vi "Begin.vi"() -> (0 "error out":errorcluster)   [LabVIEW 2014]
doc: "Called before other user functions, this VI is expected to open initial I/O refnums, load in file data, and do all program initialization. Notice that the <B>error out</B> terminal is simply used for data flow. Wiring it to other structures or subVIs ensures that this VI runs first."
uses:
  <vilib>/Rock Robotics/WPI/SafetyOutput/WPI_SafetyOutputConfigMenu.ctl
  Robot Global Data.vi
  <vilib>/Rock Robotics/WPI/DriverStation/WPI_DriverStationRobotMode2.ctl
  <vilib>/Rock Robotics/WPI/Joystick/WPI_JoystickDeviceEnum.ctl
  <vilib>/Rock Robotics/SystemInterfaces/DIO/FPGA_DIOPWMChannel.ctl
  <vilib>/Rock Robotics/SystemInterfaces/AI/FPGA_AIGyroChannel.ctl
  <vilib>/Rock Robotics/SystemInterfaces/Typedef/FPGA_TypedefAnalogModuleForGyro.ctl
  <vilib>/Rock Robotics/WPI/Counter/WPI_CounterDigitalInputToDigitalSource.vi
  <vilib>/Rock Robotics/SystemInterfaces/DIO/FPGA_DIOChannel.ctl
  <vilib>/Rock Robotics/WPI/Encoder/WPI_EncoderType.ctl
  <vilib>/Rock Robotics/SystemInterfaces/DIO/FPGA_DIORelayChannel.ctl
  <vilib>/Rock Robotics/WPI/Relay/WPI_RelayDirection.ctl
  <vilib>/Rock Robotics/SystemInterfaces/Typedef/FPGA_TypedefDigitalModule.ctl
  <vilib>/Rock Robotics/WPI/MotorControl/WPI_MotorControlOpen Victor.vi
  <vilib>/Rock Robotics/WPI/Relay/WPI_RelayValue.ctl
  <vilib>/Rock Robotics/WPI/RobotDrive/WPI_RobotDriveOpen4MotorWithTalon.vi
  <vilib>/Rock Robotics/SystemInterfaces/AI/FPGA_AIChannel.ctl
panel:
  out "error out 7":errorcluster
  out "error out 6":errorcluster
  out "error out 5":errorcluster
  out "error out 4":errorcluster
  out "error out 3":errorcluster
  out "error out 2":errorcluster
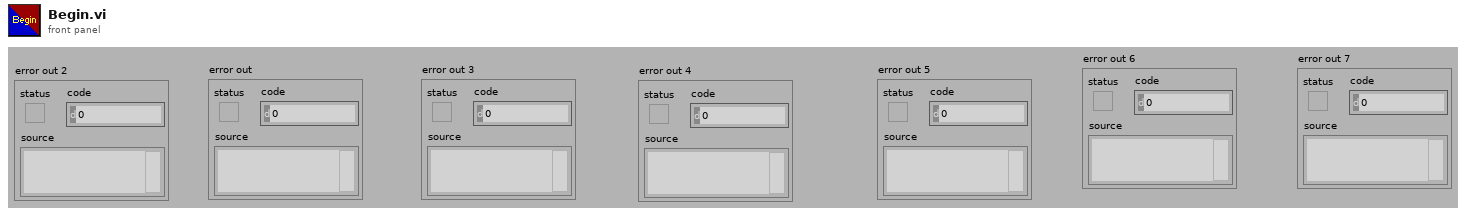
[diagram p1: front panel]
types:
  T1 = typedef "FPGA_AIChannel.ctl" = enum8{"AI 1", "AI 2", "AI 3", "AI 4", "AI 5", "AI 6", "AI 7", "AI 8", "Invalid"}
  T2 = typedef "FPGA_DIOChannel.ctl" = enum8{"DIO 1", "DIO 2", "DIO 3", "DIO 4", "DIO 5", "DIO 6", "DIO 7", "DIO 8", "DIO 9", "DIO 10", "DIO 11", "DIO 12", "DIO 13", "DIO 14", "Invalid"}
  T3 = typedef "WPI_RelayValue.ctl" = enum16{"Off", "On", "Forward", "Reverse"}
  T4 = typedef "FPGA_TypedefDigitalModule.ctl" = enum16{"Digital Module 1", "Digital Module 2"}
  T5 = typedef "FPGA_DIORelayChannel.ctl" = enum8{"Relay 1", "Relay 2", "Relay 3", "Relay 4", "Relay 5", "Relay 6", "Relay 7", "Relay 8", "Invalid"}
  T6 = typedef "FPGA_DIOPWMChannel.ctl" = enum8{"PWM 1", "PWM 2", "PWM 3", "PWM 4", "PWM 5", "PWM 6", "PWM 7", "PWM 8", "PWM 9", "PWM 10", "Invalid"}
  T7 = typedef "WPI_RelayDirection.ctl" = enum16{"Both directions", "Forward only", "Reverse only"}
  T8 = typedef "WPI_EncoderType.ctl" = enum16{"1x", "2x", "4x"}
  T9 = typedef "WPI_JoystickDeviceEnum.ctl" = enum16{"USB 1", "USB 2", "USB 3", "USB 4", "Kinect 1", "Kinect 2"}
  T10 = typedef "FPGA_TypedefAnalogModuleForGyro.ctl" = enum16{"Analog Module 1"}
  T11 = typedef "FPGA_AIGyroChannel.ctl" = enum8{"AI 1", "AI 2", "Invalid"}
  T12 = typedef "WPI_DriverStationRobotMode2.ctl" = enum16{"Autonomous Disabled", "Autonomous Enabled", "Teleop Disabled", "Teleop Enabled", "Timeout", "Finish", "Test Disabled", "Test Enabled"}
  T13 = typedef "WPI_SafetyOutputConfigMenu.ctl" = enum16{"Enable", "Disable"}
  T14 = typedef "WPI_AnalogChannelDevRef.ctl" = cluster{"DevStatus":errorcluster, "Analog Module":T15, "Analog Channel":T1}
  T15 = typedef "FPGA_TypedefAnalogModule.ctl" = enum16{"Analog Module 1", "Analog Module 2"}
  T16 = typedef "WPI_DigitalInputDevRef.ctl" = cluster{"DevStatus":errorcluster, "DIO Channel":T2, "Digital Module":T4}
  T17 = typedef "WPI_JoystickDevRef.ctl" = cluster{"Device":T9}
  T18 = typedef "WPI_MotorControlDeviceRef.ctl" = cluster{"DeviceStatus":errorcluster, "Type":enum16{"PWM", "CAN"}, "PWM":cluster{"Digital Module":T4, "PWM Channel":T6, "DeadBand":T19}, "CAN":cluster{"Device Number":u8, "Control Mode":T20, "Semaphore":T21, "Max Vout":dbl}, "Invert":bool, "TransformRef":T22, "InvTransformRef":T22}
  T19 = typedef "WPI_PWMDeadband.ctl" = cluster{"Name":string, "maxPositivePwm":i32, "minPositivePwm":i32, "centerPwm":i32, "maxNegativePwm":i32, "minNegativePwm":i32, "angularRange":u16}
  T20 = typedef "WPI_CANJaguar_ControlMode.ctl" = enum8{"Percent VBus", "Current", "Speed", "Position", "Voltage"}
  T21 = typedef "Semaphore RefNum" = refnum<k1>
  T22 = typedef "WPI_PWMTransform_ConPane.ctl" = refnum<vi>
  T23 = typedef "WPI_RelayDevRef.ctl" = cluster{"DevStatus":errorcluster, "Relay Channel":T5, "Digital Module":T4, "Relay Direction":T7}
  T24 = typedef "FPGA_CounterEncoderSourceConvertionLVSourceType.ctl" = cluster{"DevStatus":errorcluster, "AnalogTriggerMode?":bool, "DigitalMode":cluster{"Digital Module":T4, "DIO Channel":T25}, "AnalogTriggerMode":cluster{"AnalogTriggerIndex":T26, "OutputType":T27}}
  T25 = typedef "FPGA_DIODigitalSourceChannel.ctl" = enum8{"DIO 1", "DIO 2", "DIO 3", "DIO 4", "DIO 5", "DIO 6", "DIO 7", "DIO 8", "DIO 9", "DIO 10", "DIO 11", "DIO 12", "DIO 13", "DIO 14", "Disabled"}
  T26 = typedef "FPGA_AnalogTriggerIndex.ctl" = enum8{"Trig 0", "Trig 1", "Trig 2", "Trig 3", "Trig 4", "Trig 5", "Trig 6", "Trig 7", "Invalid"}
  T27 = typedef "FPGA_AnalogTriggerOutType.ctl" = enum16{"InWindow", "TriggerState", "Rising", "Falling"}
  T28 = typedef "WPI_RobotDriveDevRef.ctl" = cluster{"DevStatus":errorcluster, "Motors[]":T18[], "Square Inputs":bool, "Max Output":dbl, "Isochronous":bool}
  T29 = typedef "WPI_CompressorDevRef.ctl" = cluster{"DevStatus":errorcluster, "DigitalInputDevRef":T16, "RelayDevRef":T23}
  T30 = typedef "WPI_GyroDevRef.ctl" = cluster{"DevStatus":errorcluster, "Analog Module":T15, "Analog Channel":T1, "Offset":dbl, "Gain (VoltsPerDegree/Second)":dbl}
  T31 = typedef "WPI_EncoderDevRef.ctl" = cluster{"DevStatus":errorcluster, "EncoderIndex":T32, "CounterIndex":T33, "DistancePerCount":dbl, "Decoding Type":T8}
  T32 = typedef "FPGA_EncoderIdx.ctl" = enum8{"Enc 0", "Enc 1", "Enc 2", "Enc 3", "Invalid"}
  T33 = typedef "FPGA_CounterCtrSystemIndex.ctl" = enum8{"Ctr 0", "Ctr 1", "Ctr 2", "Ctr 3", "Ctr 4", "Ctr 5", "Ctr 6", "Ctr 7", "Invalid"}
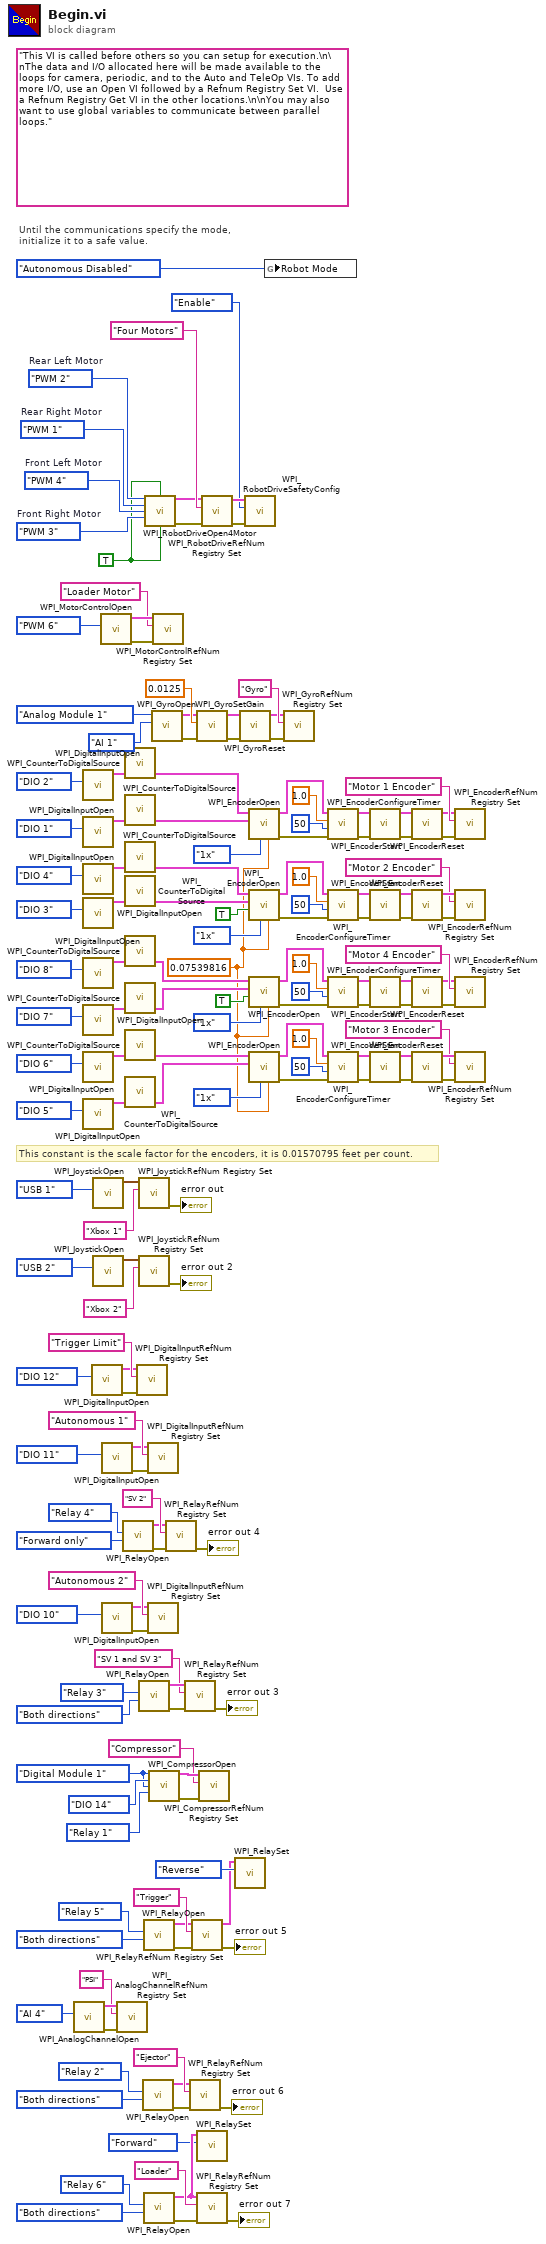
[diagram p0: block diagram]
diagram:
  w19 = FPGA_TypedefDigitalModule."Digital Module 1" ("Pressure Switch Digital Module (Module 1)")
  w22 = TRUE
  w10 = 0.07539816 ("DistancePerCount")
  w156 = FPGA_DIOPWMChannel."PWM 3"  # Front Right Motor
  w157 = FPGA_DIOPWMChannel."PWM 4"  # Front Left Motor
  w158 = FPGA_DIOPWMChannel."PWM 1"  # Rear Right Motor
  w159 = FPGA_DIOPWMChannel."PWM 2"  # Rear Left Motor
  (unwired) "This VI is called before others so you can setup for execution.\n\nThe data and I/O allocated here will be made available to the loops for camera, periodic, and to the Auto and TeleOp VIs. To add more I/O, use an Open VI followed by a Refnum Registry Set VI.  Use a Refnum Registry Get VI in the other locations.\n\nYou may also want to use global variables to communicate between parallel loops."
  # "This constant is the scale factor for the encoders, it is 0.01570795 feet per count."
  # "Until the communications specify the mode,\ninitialize it to a safe value."
  n1 = call <vilib>:"WPI_AnalogChannelOpen.vi"("Analog Channel"=FPGA_AIChannel."AI 4") -> ("error out"=w4:errorcluster, "AIDeviceRef"=w3:T14)  [unwired: 9 in]
  n2 = call <vilib>:"WPI_DigitalInputOpen.vi"("DIO Channel"=FPGA_DIOChannel."DIO 2") -> ("DigitalInputDevRef"=w63:T16)  [unwired: 2 in, 8 out]
  n3 = call <vilib>:"WPI_DigitalInputOpen.vi"("DIO Channel"=FPGA_DIOChannel."DIO 1") -> ("DigitalInputDevRef"=w62:T16)  [unwired: 2 in, 8 out]
  n4 = call <vilib>:"WPI_DigitalInputOpen.vi"("DIO Channel"=FPGA_DIOChannel."DIO 4") -> ("DigitalInputDevRef"=w94:T16)  [unwired: 2 in, 8 out]
  n5 = call <vilib>:"WPI_DigitalInputOpen.vi"("DIO Channel"=FPGA_DIOChannel."DIO 3") -> ("DigitalInputDevRef"=w95:T16)  [unwired: 2 in, 8 out]
  n6 = call <vilib>:"WPI_DigitalInputOpen.vi"("DIO Channel"=FPGA_DIOChannel."DIO 8") -> ("DigitalInputDevRef"=w99:T16)  [unwired: 2 in, 8 out]
  n7 = call <vilib>:"WPI_DigitalInputOpen.vi"("DIO Channel"=FPGA_DIOChannel."DIO 7") -> ("DigitalInputDevRef"=w98:T16)  [unwired: 2 in, 8 out]
  n8 = call <vilib>:"WPI_DigitalInputOpen.vi"("DIO Channel"=FPGA_DIOChannel."DIO 6") -> ("DigitalInputDevRef"=w131:T16)  [unwired: 2 in, 8 out]
  n9 = call <vilib>:"WPI_DigitalInputOpen.vi"("DIO Channel"=FPGA_DIOChannel."DIO 5") -> ("DigitalInputDevRef"=w132:T16)  [unwired: 2 in, 8 out]
  n10 = call <vilib>:"WPI_DigitalInputOpen.vi"("DIO Channel"=FPGA_DIOChannel."DIO 12") -> ("error out"=w6:errorcluster, "DigitalInputDevRef"=w7:T16)  [unwired: 2 in, 7 out]
  n11 = call <vilib>:"WPI_JoystickOpen.vi"("JoystickDevice"=WPI_JoystickDeviceEnum."USB 1") -> ("JoystickDevRef"=w58:T17)  [unwired: 10 in]
  n12 = call <vilib>:"WPI_JoystickOpen.vi"("JoystickDevice"=WPI_JoystickDeviceEnum."USB 2") -> ("JoystickDevRef"=w137:T17)  [unwired: 10 in]
  n13 = call-poly <vilib>:"WPI_MotorControlOpen.vi"("PWM Channel"=FPGA_DIOPWMChannel."PWM 6") -> ("error out"=w24:errorcluster, "MotorControlDeviceRef"=w25:T18)  [unwired: 9 in]
  n14 = call <vilib>:"WPI_DigitalInputOpen.vi"("DIO Channel"=FPGA_DIOChannel."DIO 11") -> ("error out"=w28:errorcluster, "DigitalInputDevRef"=w30:T16)  [unwired: 2 in, 7 out]
  n15 = call <vilib>:"WPI_DigitalInputOpen.vi"("DIO Channel"=FPGA_DIOChannel."DIO 10") -> ("error out"=w27:errorcluster, "DigitalInputDevRef"=w29:T16)  [unwired: 2 in, 7 out]
  n16 = call <vilib>:"WPI_AnalogChannelRefNum Registry Set.vi"("error in (no error)"=w4, "refnum name"="PSI", "AIDeviceRef"=w3) -> ()  [unwired: 7 in, 2 out]
  n17 = call <vilib>:"WPI_RelayOpen.vi"("Relay Direction"=WPI_RelayDirection."Forward only", "Relay Channel"=FPGA_DIORelayChannel."Relay 4") -> ("error out"=w51:errorcluster, "RelayDevRef"=w52:T23)  [unwired: 8 in]
  n18 = call-poly <vilib>:"WPI_CounterToDigitalSource.vi"("DigitalInputDevRef"=w63) -> ("Digital Source"=w64:T24)  [unwired: 6 out]
  n19 = call-poly <vilib>:"WPI_CounterToDigitalSource.vi"("DigitalInputDevRef"=w62) -> ("Digital Source"=w61:T24)  [unwired: 6 out]
  n20 = call-poly <vilib>:"WPI_CounterToDigitalSource.vi"("DigitalInputDevRef"=w94) -> ("Digital Source"=w93:T24)  [unwired: 6 out]
  n21 = call-poly <vilib>:"WPI_CounterToDigitalSource.vi"("DigitalInputDevRef"=w95) -> ("Digital Source"=w96:T24)  [unwired: 6 out]
  n22 = call-poly <vilib>:"WPI_CounterToDigitalSource.vi"("DigitalInputDevRef"=w99) -> ("Digital Source"=w100:T24)  [unwired: 6 out]
  n23 = call-poly <vilib>:"WPI_CounterToDigitalSource.vi"("DigitalInputDevRef"=w98) -> ("Digital Source"=w97:T24)  [unwired: 6 out]
  n24 = call-poly <vilib>:"WPI_CounterToDigitalSource.vi"("DigitalInputDevRef"=w131) -> ("Digital Source"=w130:T24)  [unwired: 6 out]
  n25 = call-poly <vilib>:"WPI_CounterToDigitalSource.vi"("DigitalInputDevRef"=w132) -> ("Digital Source"=w133:T24)  [unwired: 6 out]
  n26 = call <vilib>:"WPI_DigitalInputRefNum Registry Set.vi"("error in (no error)"=w6, "refnum name"="Trigger Limit", "DigitalInputDevRef"=w7) -> ()  [unwired: 7 in, 2 out]
  n27 = call <vilib>:"WPI_JoystickRefNum Registry Set.vi"("refnum name"="Xbox 1", "JoystickDevRef"=w58) -> ("error out"=→"error out":errorcluster)  [unwired: 8 in, 1 out]
  n28 = call <vilib>:"WPI_JoystickRefNum Registry Set.vi"("refnum name"="Xbox 2", "JoystickDevRef"=w137) -> ("error out"=→"error out 2":errorcluster)  [unwired: 8 in, 1 out]
  n29 = call <vilib>:"WPI_RelayOpen.vi"("Relay Direction"=WPI_RelayDirection."Both directions", "Relay Channel"=FPGA_DIORelayChannel."Relay 3") -> ("error out"=w144:errorcluster, "RelayDevRef"=w143:T23)  [unwired: 8 in]
  n30 = call <vilib>:"WPI_RelayOpen.vi"("Relay Direction"=WPI_RelayDirection."Both directions", "Relay Channel"=FPGA_DIORelayChannel."Relay 2") -> ("error out"=w40:errorcluster, "RelayDevRef"=w41:T23)  [unwired: 8 in]
  n31 = call <vilib>:"WPI_RelayOpen.vi"("Relay Direction"=WPI_RelayDirection."Both directions", "Relay Channel"=FPGA_DIORelayChannel."Relay 5") -> ("error out"=w50:errorcluster, "RelayDevRef"=w14:T23)  [unwired: 8 in]
  n32 = call <vilib>:"WPI_RelayOpen.vi"("Relay Direction"=WPI_RelayDirection."Both directions", "Relay Channel"=FPGA_DIORelayChannel."Relay 6") -> ("error out"=w39:errorcluster, "RelayDevRef"=w12:T23)  [unwired: 8 in]
  n33 = call-poly <vilib>:"WPI_RobotDriveOpen4Motor.vi"("Rear Left Motor"=w159, "Rear Right Motor Inverted"=w22, "Rear Right Motor"=w158, "Front Left Motor"=w157, "Front Right Motor"=w156, "Front Right Motor Inverted"=w22) -> ("RobotDriveDevRef"=w1:T28, "error out"=w163:errorcluster)  [unwired: 8 in]
  n34 = call <vilib>:"WPI_DigitalInputRefNum Registry Set.vi"("error in (no error)"=w28, "refnum name"="Autonomous 1", "DigitalInputDevRef"=w30) -> ()  [unwired: 7 in, 2 out]
  n35 = call <vilib>:"WPI_DigitalInputRefNum Registry Set.vi"("error in (no error)"=w27, "refnum name"="Autonomous 2", "DigitalInputDevRef"=w29) -> ()  [unwired: 7 in, 2 out]
  n36 = call <vilib>:"WPI_CompressorOpen.vi"("Pressure Switch Digital Module (Module 1)"=w19, "Pressure Switch DIO Channel"=FPGA_DIOChannel."DIO 14", "Relay Digital Module (Module 1)"=w19, "Relay Channel"=FPGA_DIORelayChannel."Relay 1") -> ("CompressorDevRef"=w17:T29, "error out"=w18:errorcluster)  [unwired: 10 in]
  n37 = call <vilib>:"WPI_GyroOpen.vi"("Analog Channel"=FPGA_AIGyroChannel."AI 1" ("Channel"), "Analog Module (Module 1)"=FPGA_TypedefAnalogModuleForGyro."Analog Module 1" ("Analog Module")) -> ("error out"=w150:errorcluster, "GyroDevRef"=w151:T30)  [unwired: 4 in, 4 out]
  n38 = call <vilib>:"WPI_MotorControlRefNum Registry Set.vi"("error in (no error)"=w24, "refnum name"="Loader Motor", "MotorControlDevRef"=w25) -> ()  [unwired: 7 in, 2 out]
  n39 = call <vilib>:"WPI_RelayRefNum Registry Set.vi"("error in (no error)"=w51, "refnum name"="SV 2", "RelayDevRef"=w52) -> ("error out"=→"error out 4":errorcluster)  [unwired: 7 in, 1 out]
  n40 = call <vilib>:"WPI_RelayRefNum Registry Set.vi"("error in (no error)"=w144, "refnum name"="SV 1 and SV 3", "RelayDevRef"=w143) -> ("error out"=→"error out 3":errorcluster)  [unwired: 7 in, 1 out]
  n41 = call <vilib>:"WPI_RelayRefNum Registry Set.vi"("error in (no error)"=w40, "refnum name"="Ejector", "RelayDevRef"=w41) -> ("error out"=→"error out 6":errorcluster)  [unwired: 7 in, 1 out]
  n42 = call <vilib>:"WPI_RelayRefNum Registry Set.vi"("error in (no error)"=w50, "refnum name"="Trigger", "RelayDevRef"=w14) -> ("error out"=→"error out 5":errorcluster, "RelayDevRef"=w13:T23)  [unwired: 7 in]
  n43 = call <vilib>:"WPI_GyroSetGain.vi"("error in (no error)"=w150, "Gain (VoltsPerDegree/Second)"=0.0125, "GyroDevRef"=w151) -> ("error out"=w148:errorcluster, "GyroDevRef"=w149:T30)  [unwired: 7 out]
  n44 = call <vilib>:"WPI_RelaySet.vi"("RelayValue"=WPI_RelayValue."Forward", "RelayDevRef"=w12) -> ()  [unwired: 8 in, 2 out]
  n45 = call <vilib>:"WPI_RelayRefNum Registry Set.vi"("error in (no error)"=w39, "refnum name"="Loader", "RelayDevRef"=w12) -> ("error out"=→"error out 7":errorcluster)  [unwired: 7 in, 1 out]
  n46 = call <vilib>:"WPI_CompressorRefNum Registry Set.vi"("error in (no error)"=w18, "refnum name"="Compressor", "CompressorDevRef"=w17) -> ()  [unwired: 7 in, 2 out]
  n47 = call <vilib>:"WPI_RobotDriveRefNum Registry Set.vi"("error in (no error)"=w163, "refnum name"="Four Motors", "RobotDriveDevRef"=w1) -> ("error out"=w145:errorcluster, "RobotDriveDevRef"=w162:T28)  [unwired: 7 out]
  n48 = call <vilib>:"WPI_RelaySet.vi"("RelayValue"=WPI_RelayValue."Reverse", "RelayDevRef"=w13) -> ()  [unwired: 8 in, 2 out]
  n49 = call <vilib>:"WPI_GyroReset.vi"("error in (no error)"=w148, "GyroDevRef"=w149) -> ("error out"=w146:errorcluster, "GyroDevRef"=w147:T30)  [unwired: 8 out]
  n50 = call <vilib>:"WPI_RobotDriveSafetyConfig.vi"("error in (no error)"=w145, "mode"=WPI_SafetyOutputConfigMenu."Enable", "RobotDriveDevRef"=w162) -> ()  [unwired: 7 in, 2 out]
  n51 = call <vilib>:"WPI_EncoderOpen.vi"("DistancePerCount"=w10, "Decoding Type"=WPI_EncoderType."1x", "BSource"=w61, "ASource"=w64) -> ("error out"=w72:errorcluster, "EncoderDevRef"=w66:T31)  [unwired: 4 in, 2 out]
  n52 = call <vilib>:"WPI_EncoderOpen.vi"("DistancePerCount"=w10, "Decoding Type"=WPI_EncoderType."1x", "Invert Direction (False)"=TRUE, "BSource"=w96, "ASource"=w93) -> ("error out"=w85:errorcluster, "EncoderDevRef"=w91:T31)  [unwired: 3 in, 2 out]
  n53 = call <vilib>:"WPI_EncoderOpen.vi"("DistancePerCount"=w10, "Decoding Type"=WPI_EncoderType."1x", "Invert Direction (False)"=TRUE, "BSource"=w97, "ASource"=w100) -> ("error out"=w108:errorcluster, "EncoderDevRef"=w102:T31)  [unwired: 3 in, 2 out]
  n54 = call <vilib>:"WPI_EncoderOpen.vi"("DistancePerCount"=w10, "Decoding Type"=WPI_EncoderType."1x", "BSource"=w133, "ASource"=w130) -> ("error out"=w122:errorcluster, "EncoderDevRef"=w128:T31)  [unwired: 4 in, 2 out]
  n55 = global write "Robot Global Data.vi" "Robot Mode"(WPI_DriverStationRobotMode2."Autonomous Disabled" ("Robot Mode")) -> ()
  n56 = call <vilib>:"WPI_GyroRefNum Registry Set.vi"("error in (no error)"=w146, "refnum name"="Gyro", "GyroDevRef"=w147) -> ()  [unwired: 7 in, 2 out]
  n57 = call <vilib>:"WPI_EncoderConfigureTimer.vi"("error in (no error)"=w72, "Number Samples to Average"=u8 50, "Minimum Rate"=1.0, "EncoderDevRef"=w66) -> ("error out"=w71:errorcluster, "EncoderDevRef"=w65:T31)  [unwired: 6 out]
  n58 = call <vilib>:"WPI_EncoderConfigureTimer.vi"("error in (no error)"=w85, "Number Samples to Average"=u8 50, "Minimum Rate"=1.0, "EncoderDevRef"=w91) -> ("error out"=w86:errorcluster, "EncoderDevRef"=w92:T31)  [unwired: 6 out]
  n59 = call <vilib>:"WPI_EncoderConfigureTimer.vi"("error in (no error)"=w108, "Number Samples to Average"=u8 50, "Minimum Rate"=1.0, "EncoderDevRef"=w102) -> ("error out"=w107:errorcluster, "EncoderDevRef"=w101:T31)  [unwired: 6 out]
  n60 = call <vilib>:"WPI_EncoderConfigureTimer.vi"("error in (no error)"=w122, "Number Samples to Average"=u8 50, "Minimum Rate"=1.0, "EncoderDevRef"=w128) -> ("error out"=w123:errorcluster, "EncoderDevRef"=w129:T31)  [unwired: 6 out]
  n61 = call <vilib>:"WPI_EncoderStart.vi"("error in (no error)"=w71, "EncoderDevRef"=w65) -> ("error out"=w70:errorcluster, "EncoderDevRef"=w69:T31)  [unwired: 8 out]
  n62 = call <vilib>:"WPI_EncoderStart.vi"("error in (no error)"=w86, "EncoderDevRef"=w92) -> ("error out"=w87:errorcluster, "EncoderDevRef"=w88:T31)  [unwired: 8 out]
  n63 = call <vilib>:"WPI_EncoderStart.vi"("error in (no error)"=w107, "EncoderDevRef"=w101) -> ("error out"=w106:errorcluster, "EncoderDevRef"=w105:T31)  [unwired: 8 out]
  n64 = call <vilib>:"WPI_EncoderStart.vi"("error in (no error)"=w123, "EncoderDevRef"=w129) -> ("error out"=w124:errorcluster, "EncoderDevRef"=w125:T31)  [unwired: 8 out]
  n65 = call <vilib>:"WPI_EncoderReset.vi"("error in (no error)"=w70, "EncoderDevRef"=w69) -> ("error out"=w73:errorcluster, "EncoderDevRef"=w74:T31)  [unwired: 8 out]
  n66 = call <vilib>:"WPI_EncoderReset.vi"("error in (no error)"=w87, "EncoderDevRef"=w88) -> ("error out"=w84:errorcluster, "EncoderDevRef"=w83:T31)  [unwired: 8 out]
  n67 = call <vilib>:"WPI_EncoderReset.vi"("error in (no error)"=w106, "EncoderDevRef"=w105) -> ("error out"=w109:errorcluster, "EncoderDevRef"=w110:T31)  [unwired: 8 out]
  n68 = call <vilib>:"WPI_EncoderReset.vi"("error in (no error)"=w124, "EncoderDevRef"=w125) -> ("error out"=w121:errorcluster, "EncoderDevRef"=w120:T31)  [unwired: 8 out]
  n69 = call <vilib>:"WPI_EncoderRefNum Registry Set.vi"("error in (no error)"=w73, "refnum name"="Motor 1 Encoder", "EncoderDevRef"=w74) -> ()  [unwired: 7 in, 2 out]
  n70 = call <vilib>:"WPI_EncoderRefNum Registry Set.vi"("error in (no error)"=w84, "refnum name"="Motor 2 Encoder", "EncoderDevRef"=w83) -> ()  [unwired: 7 in, 2 out]
  n71 = call <vilib>:"WPI_EncoderRefNum Registry Set.vi"("error in (no error)"=w109, "refnum name"="Motor 4 Encoder", "EncoderDevRef"=w110) -> ()  [unwired: 7 in, 2 out]
  n72 = call <vilib>:"WPI_EncoderRefNum Registry Set.vi"("error in (no error)"=w121, "refnum name"="Motor 3 Encoder", "EncoderDevRef"=w120) -> ()  [unwired: 7 in, 2 out]
